vi "Generate Single Overlay.vi"(8 "error in":errorcluster, 9 "Single Color":bool, 10 "Overlay":T1, 11 "BigMAQ in":refnum<class "BigMAQ.lvclass">) -> (0 "error out":errorcluster, 2 "Overlay Out":T1, 3 "BigMAQ out":refnum<class "BigMAQ.lvclass">)   [LabVIEW 2019, in "BigMAQ.lvclass"]
uses:
  BigMAQ.lvclass
  Overlay.ctl
  BigMAQ.lvclass/BigMAQ.ctl
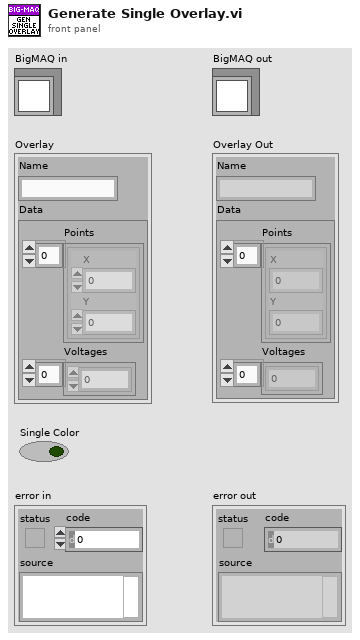
[diagram p1: front panel]
types:
  T1 = typedef "BigMAQ.lvclass/Overlay.ctl" = cluster{"Name":string, "Data":cluster{"Points":cluster{"X":dbl, "Y":dbl}[], "Voltages":dbl[]}}
  T2 = typedef "IMAQ Image.ctl" = refnum<image>
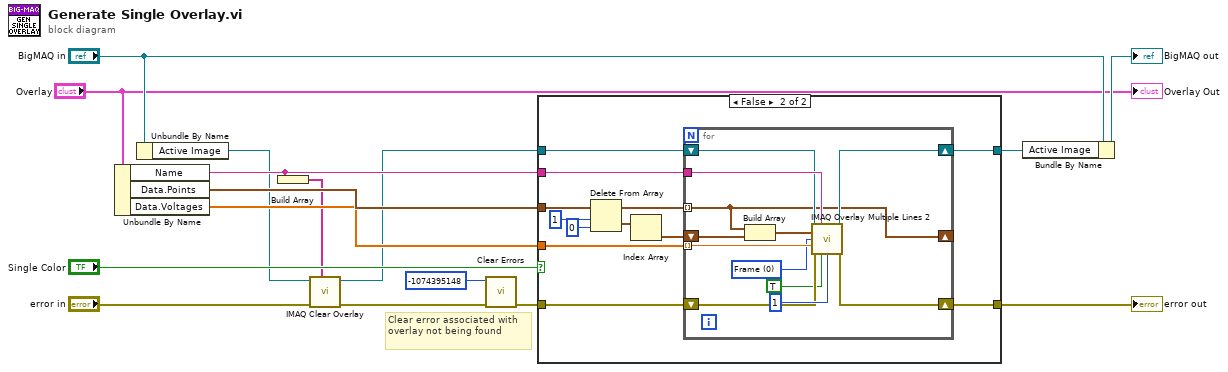
[diagram p0: block diagram]
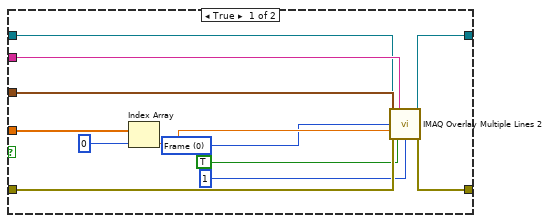
[diagram p2: hidden frame]
diagram:
  # "Clear error associated with overlay not being found"
  n1 = Unbundle By Name("Overlay") -> ("Name"=w7:string, "Data.Points"=w16:cluster{"X":dbl, "Y":dbl}[], "Data.Voltages"=w15:dbl[])
  n2 = Unbundle By Name("BigMAQ in") -> ("Active Image"=w5:T2)
  n3 = Build Array(w7) -> (w6:string[])
  n4 = call "IMAQ Clear Overlay"("Groups"=w6, "error in (no error)"="error in", "Image"=w5) -> ("error out"=w3:errorcluster, "Image Out"=w4:T2)  [unwired: 7 in]
  n5 = call <vilib>:"Clear Errors.vi"("error in (no error)"=w3, "specific error code to clear (0: all)"=-1074395148) -> ("error out"=w2:errorcluster)  [unwired: 4 in, 1 out]
  n6 = case shown="False" "Single Color" {
    tunnel: w4 -> [w20 w40]
    tunnel: w7 -> [w28 w39]
    tunnel: w2 -> [w27 w38]
    tunnel: [w21 w37] -> w9
    tunnel: w16 -> [w26 w31]
    tunnel: [w24 w36] -> w14
    tunnel: w15 -> [w23 w35]
    frame True {
      w18 = u32 0 items=["Frame", "Fill"] ("Drawing Mode (Frame)")
      n7 = Index Array(array=w23, index=0) -> (element=w22:dbl)
      n8 = call "IMAQ Overlay Multiple Lines 2"("Image"=w20, "Group"=w28, "Line End Points"=w26, "Drawing Mode (Frame)"=w18, "Color"=w22, "error in (no error)"=w27, "Maintain Width?"=TRUE, "Width"=u32 1) -> ("Image Out"=w24:T2, "error out"=w21:errorcluster)  [unwired: 6 in]
    }
    frame False {
      n9 = Delete From Array(array=w31, length=1, index=0) -> (deleted portion=w30:cluster{"X":dbl, "Y":dbl}[], array with subset deleted=w32:cluster{"X":dbl, "Y":dbl}[])
      n10 = Index Array(array=w30) -> (element=w29:cluster{"X":dbl, "Y":dbl})  [unwired: 1 in]
      n11 = for {
        tunnel: w39 -> [w52]
        tunnel: w32 -> [w42] mode=indexing
        shift-right: [w50] -> w36
        shift-left: w40 -> [w49]
        shift-right: [w48] -> w37
        shift-left: w38 -> [w47]
        tunnel: w35 -> [w45] mode=indexing
        shift-right: [w42] -> _
        shift-left: w29 -> [w43]
        w44 = u32 0 items=["Frame", "Fill"] ("Drawing Mode (Frame)")
        n12 = Build Array(w42, w43) -> (w41:cluster{"X":dbl, "Y":dbl}[])
        n13 = call "IMAQ Overlay Multiple Lines 2"("Image"=w49, "Group"=w52, "Line End Points"=w41, "Drawing Mode (Frame)"=w44, "Color"=w45, "error in (no error)"=w47, "Maintain Width?"=TRUE, "Width"=u32 1) -> ("Image Out"=w50:T2, "error out"=w48:errorcluster)  [unwired: 6 in]
      }
    }
  }
  "error out" <- w9
  n14 = Bundle By Name(cluster="BigMAQ in", "Active Image"=w14) -> (→"BigMAQ out":refnum<class "BigMAQ.lvclass">)
  "Overlay Out" <- "Overlay"
